vi "DueDACtoAURORA_MM.vi"() -> ()   [LabVIEW 2011]
uses:
  <vilib>/rvi/FXPMathLib/FxpSub/subVIs/nifxpmath_Sub_SimConfig.ctl
  <vilib>/fxp/LVFixedPointQuantizationPolicyTypeDef.ctl
  <vilib>/fxp/LVFixedPointOverflowPolicyTypeDef.ctl
  <vilib>/rvi/FXPMathLib/FxpDiv/subVIs/nifxpmath_Div_SimConfig.ctl
  <vilib>/rvi/interface/RandomDataEmulation/nirviRandomDataFPGAFIFO.vi
  <vilib>/rvi/interface/RandomDataEmulation/niFpgaRandomDataHandleErrors.vi
  <vilib>/rvi/eio/common/nirviEmuTemplateMethod_errors.vi
  <vilib>/rvi/FXPMathLib/FxpSub/simVIs/DllFxpSubTemp_sub.vi
  <vilib>/rvi/FXPMathLib/FxpDiv/simVIs/DllFxpDivTemp_sub.vi
  <vilib>/rvi/DataTransferAndStorage/Container/XNode/niFpgaContainer.xnode
  <vilib>/rvi/interface/RandomDataEmulation/nirviRandomDataFpgaReadWriteTemplate.vi
  <vilib>/eio/EIONode/EIONode.xnode
  <vilib>/rvi/FXPMathLib/FxpAdd/XNode/nifxpmath_Add.xnode
  <vilib>/rvi/FXPMathLib/FxpMul/XNode/nifxpmath_Multiplier.xnode
  <vilib>/rvi/Analysis/measure/butterworth/XNode/niFpgaButterworthFilter.xnode
  <vilib>/rvi/Analysis/common/FxpNativeNode/niFpgaFxpNative.xnode
  <vilib>/rvi/FXPMathLib/FxpSub/XNode/nifxpmath_Sub.xnode
  <vilib>/rvi/FXPMathLib/FxpDiv/XNode/nifxpmath_Div.xnode
  <vilib>/rvi/FXPMathLib/sim/FxpSim.dll
panel:
  in  "N or torque (V)\noutput":bool
  out "non offset torque":fxp<+/-,23,1>
  out "torque to R2":fxp<+/-,23,2>
  out "torque (Nm)":fxp<+/-,23,2>
  in  "torque offset (V)":fxp<+/-,23,2>
  in  "V/Nm":fxp<+/-,21,6>=-17.579986572265625
  out "MM force":fxp<+/-,20,4>
  out "FV gain":fxp<+/-,17,2>
  out "ML/s":fxp<+/-,20,11>
  in  "Velocity filter settings":i16(ring)=1 items=["No filter", "20 Hz Lowpass", "40 Hz  Lowpass", "60 Hz Lowpass"]
  in  "V to ML":fxp<+,15,3>=0.14501953125
  out "length out reset":fxp<+/-,17,10>
  in  "Reset Mode":bool=TRUE
  out "filtered force":fxp<+/-,30,9>
  out "raw force":fxp<+/-,26,5>
  in  "length offset (V)":fxp<+/-,12,5>
  in  "Gandalf volts/rad":fxp<+/-,17,6>=12.33984375
  in  "abs length limit (V)":fxp<+/-,12,5>=9.0
  out "offset dac":fxp<+/-,27,6>
  out "Mujoco\nmuscle length\nscaled 0.145 ML/V":fxp<+/-,26,5>
  in  "DU dac gain":fxp<+/-,16,2>=1.25
  in  "DU dac\noffset":fxp<+/-,16,1>=-0.555999755859375
  out "from DUE dac0":fxp<+/-,26,5>
  out "loop time (ticks)":u32
  out "length out (V)":fxp<+/-,17,10>
  in  "Reset":bool=TRUE
  in  "Timeout":i32
  out "Full Flag\nTimed Out?":bool
  # "NOTE: Dac output has\nto be truncated so only\n2 digits of precision due\nto uncertainty of the rest."
  # "Convert 0-2.2V output to full muscle strain 0.32 ML\nEstimated by muscle dL required to make joints 180"
  # "Gain and offset to compensate for limitations of Arduino DUE\nDAC"
  # "<--Negate depending\non R2D2 direction needed"
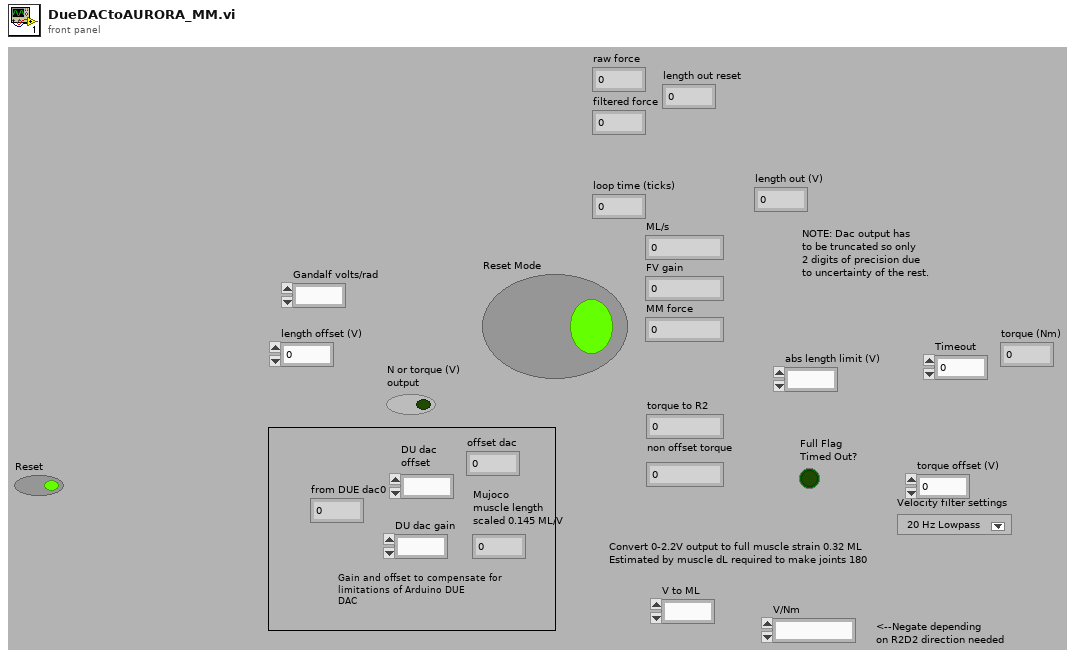
[diagram p1: front panel]
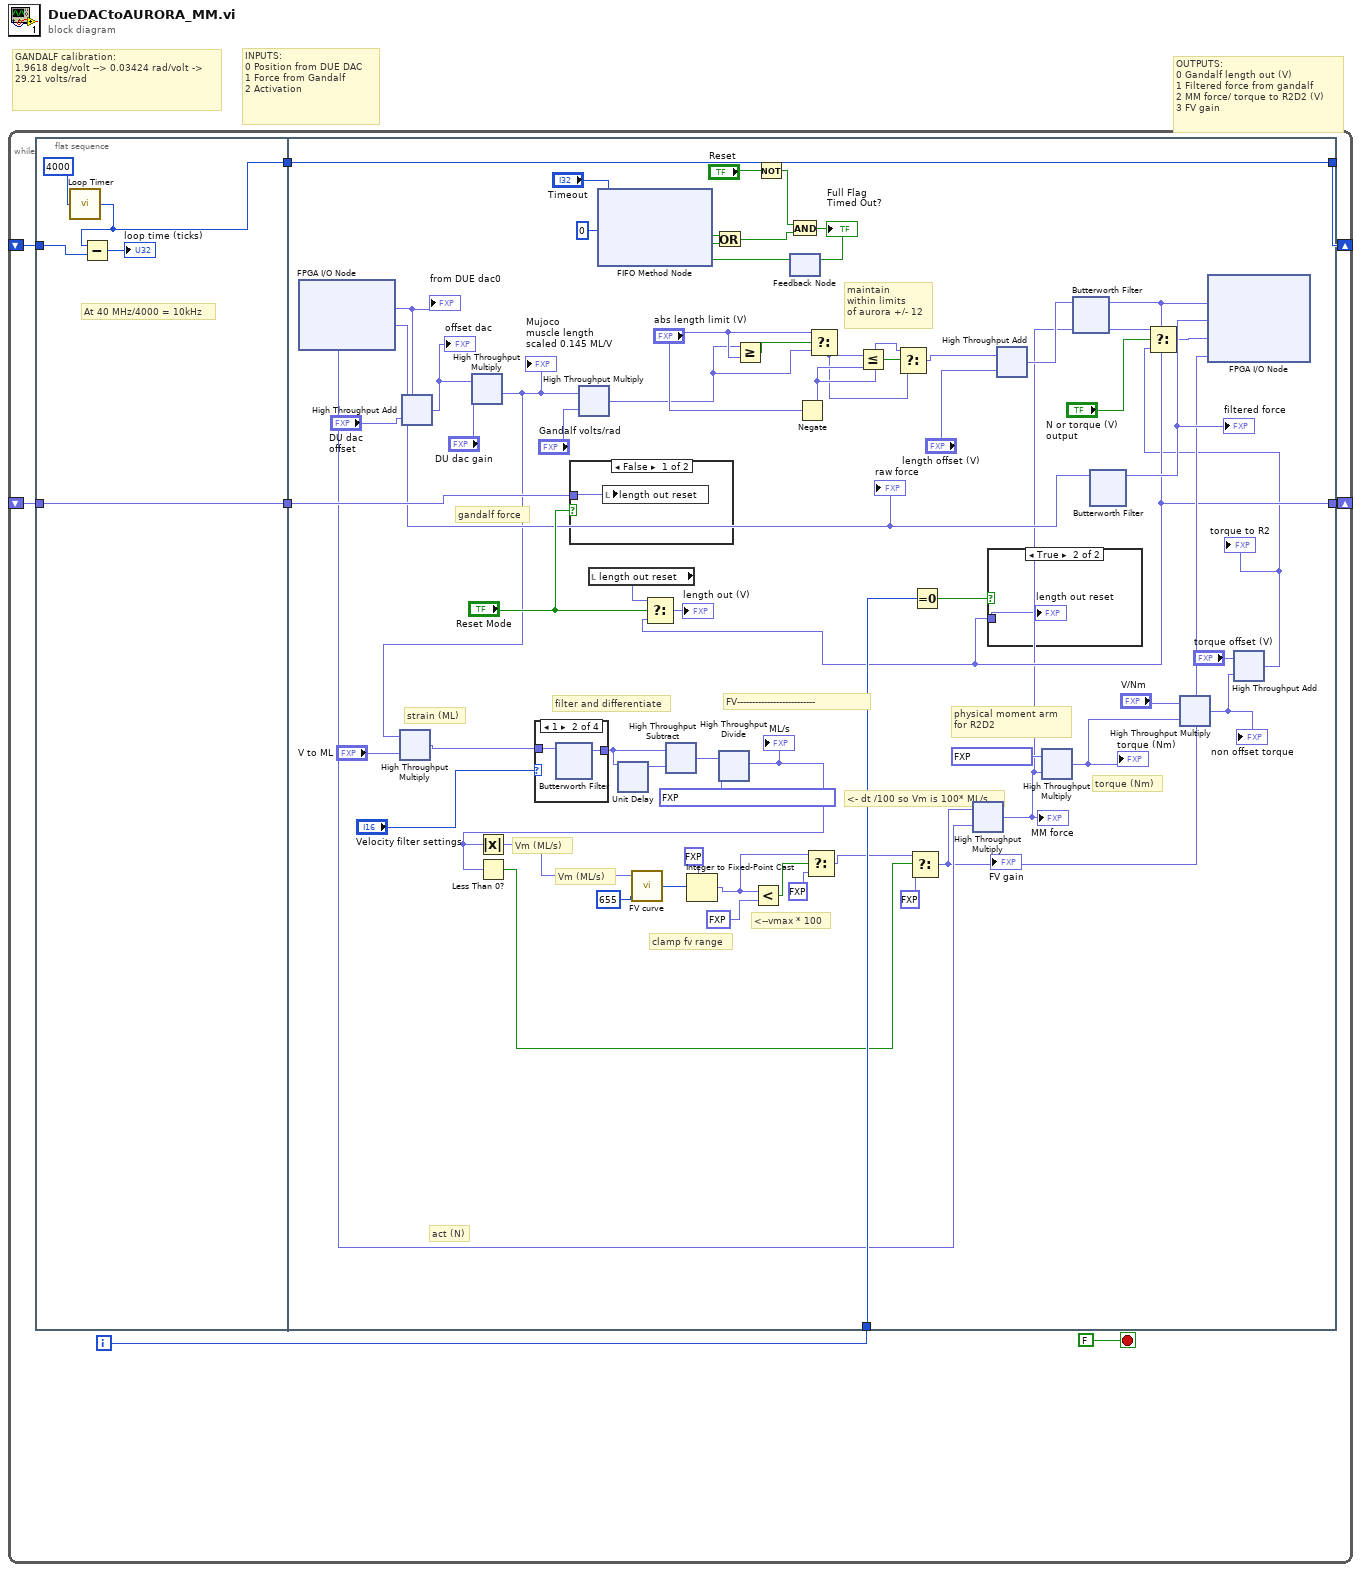
[diagram p0: block diagram]
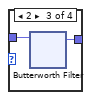
[diagram p3: hidden frame]
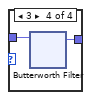
[diagram p4: hidden frame]
diagram:
  # "GANDALF calibration:\n1.9618 deg/volt --> 0.03424 rad/volt ->\n29.21 volts/rad"
  # "INPUTS:\n0 Position from DUE DAC\n1 Force from Gandalf\n2 Activation"
  # "OUTPUTS:\n0 Gandalf length out (V)\n1 Filtered force from gandalf\n2 MM force/ torque to R2D2 (V)\n3 FV gain"
  n1 = while {
    shift-right: [w7] -> _
    shift-left: _ -> [w5]
    shift-right: [w4] -> _
    shift-left: _ -> [w2]
    i -> [w1]
    stop <- FALSE stop-if-true
    n2 = flat-sequence {
      tunnel: [w11] -> w6
      tunnel: w5 -> [w12]
      tunnel: [w9] -> w3
      tunnel: w2 -> [w9]
      tunnel: [w69] -> w7
      tunnel: w6 -> [w69]
      tunnel: [w18] -> w4
      tunnel: w3 -> [w54]
      tunnel: w1 -> [w50]
      frame #0 {
        # "At 40 MHz/4000 = 10kHz"
        n3 = call "Loop Timer"("Count(Ticks)"=u32 4000) -> ("Tick Count(Ticks)"=w11:u32)
        n4 = Subtract(x=w11, y=w12) -> (x-y=→"loop time (ticks)":u32)
      }
      frame #1 {
        # "<--vmax * 100"
        # "clamp fv range"
        # "Vm (ML/s)"
        # "<- dt /100 so Vm is 100* ML/s"
        # "physical moment arm\nfor R2D2"
        # "torque (Nm)"
        # "gandalf force"
        # "act (N)"
        # "filter and differentiate"
        # "FV--------------------------"
        # "Vm (ML/s)"
        # "strain (ML)"
        # "maintain \nwithin limits\nof aurora +/- 12"
        n5 = xnode "FPGA I/O Node"() -> ("Mod2/AI0"=w20:fxp<+/-,26,5>, "Mod2/AI1"=w48:fxp<+/-,26,5>, "Mod2/AI2"=w27:fxp<+/-,26,5>)  [unwired: 3 in, 3 out]
        "from DUE dac0" <- w20
        "raw force" <- w48
        n6 = xnode "High Throughput Add"("x"=w20, "y"="DU dac\noffset") -> ("x+y"=w60:fxp<+/-,26,5>)
        "offset dac" <- w60
        n7 = xnode "High Throughput Multiply"("x"=w60, "y"="DU dac gain") -> ("x*y"=w38:fxp<+/-,26,5>)
        "Mujoco\nmuscle length\nscaled 0.145 ML/V" <- w38
        n8 = xnode "High Throughput Multiply"("x"=w38, "y"="V to ML") -> ("x*y"=w39:fxp<+/-,25,2>)
        n9 = case shown="1" "Velocity filter settings" {
          tunnel: [w91 w93 w102 w111] -> w44
          tunnel: w39 -> [w91 w92 w101 w110]
          frame 0, Default {
            # "no filter"
          }
          frame 1 {
            n10 = xnode "Butterworth Filter"("input data"=w92) -> ("output data"=w93:fxp<+/-,25,2>)  [unwired: 2 in]
          }
          frame 2 {
            n11 = xnode "Butterworth Filter"("input data"=w101) -> ("output data"=w102:fxp<+/-,25,2>)  [unwired: 2 in]
          }
          frame 3 {
            n12 = xnode "Butterworth Filter"("input data"=w110) -> ("output data"=w111:fxp<+/-,25,2>)  [unwired: 2 in]
          }
        }
        n13 = case shown="False" "Reset Mode" {
          tunnel: w54 -> [w184 _]
          frame False {
            n14 = local write "length out reset"(w184) -> ()
          }
          frame True {
          }
        }
        n15 = xnode "High Throughput Multiply"("x"=w38, "y"="Gandalf volts/rad") -> ("x*y"=w58:fxp<+/-,12,5>)
        n16 = local read "length out reset"() -> (w49:fxp<+/-,17,10>)
        n17 = xnode ("FIFO Method Node")("Element"=i16 0, "Timeout"="Timeout") -> ("Timed Out?"=w75:bool)  [unwired: 1 in, 1 out]
        n18 = xnode ("Unit Delay")("input"=w44) -> ("output"=w46:fxp<+/-,25,2>)  [unwired: 2 in]
        n19 = xnode "High Throughput Subtract"("x"=w44, "y"=w46) -> ("x-y"=w43:fxp<+/-,30,1>)
        n20 = xnode "High Throughput Divide"("x"=w43, "y"=fxp<+/-,32,1> 9.997747838497162e-07) -> ("x/y"=w42:fxp<+/-,20,11>)
        "ML/s" <- w42
        n21 = Absolute Value(x=w42) -> (abs(x)=w29:fxp<+,20,11>)
        n22 = Less Than 0?(x=w42) -> (x < 0?=w41:bool)
        n23 = call "FV curve"("address"=w29, "fractional index (x 2^16)"=u16 655) -> ("data out"=w31:i16)  [unwired: 7 in]
        n24 = Integer to Fixed-Point Cast(fixed-point type=fxp<+/-,16,1> 0.0 ("fixed-point"), integer=w31) -> (fixed-point=w23:fxp<+/-,16,1>)
        n25 = Greater Or Equal?(x=w58, y="abs length limit (V)") -> (x >= y?=w67:bool)
        n26 = Less?(x=w23, y=fxp<+/-,20,11> 900.0 ("x/y")) -> (x < y?=w24:bool)
        n27 = Not(x="Reset") -> (.not. x?=w73:bool)
        n28 = feedback #1() -> (w70:bool)  [unwired: 1 in]
        n29 = Or(x=w70, y=w75) -> (x .or. y?=w72:bool)
        n30 = And(x=w73, y=w72) -> (x .and. y?=w71:bool)
        "Full Flag\nTimed Out?" <- w71
        n31 = feedback-in #1(w71) -> ()
        n32 = Negate(x="abs length limit (V)") -> (-x=w64:fxp<+/-,13,6>)
        n33 = Select(t=w23, s=w24, f=fxp<+/-,16,1> 0.0) -> (s? t:f=w21:fxp<+/-,16,1>)
        n34 = Select(t="abs length limit (V)", s=w67, f=w58) -> (s? t:f=w63:fxp<+/-,12,5>)
        n35 = Less Or Equal?(x=w63, y=w64) -> (x <= y?=w65:bool)
        n36 = Select(t=w64, s=w65, f=w63) -> (s? t:f=w56:fxp<+/-,13,6>)
        n37 = Select(t=w21, s=w41, f=fxp<+/-,17,2> 1.0) -> (s? t:f=w26:fxp<+/-,17,2>)
        "FV gain" <- w26
        n38 = Equal To 0?(x=w50) -> (x = 0?=w51:bool)
        n39 = xnode "High Throughput Multiply"("x"=w26, "y"=w27) -> ("x*y"=w15:fxp<+/-,20,4>)
        "MM force" <- w15
        n40 = xnode "High Throughput Add"("x"=w56, "y"="length offset (V)") -> ("x+y"=w19:fxp<+/-,12,5>)
        n41 = xnode "High Throughput Multiply"("x"=fxp<+/-,21,6> 0.02001953125, "y"=w15) -> ("x*y"=w35:fxp<+/-,23,2>)
        "torque (Nm)" <- w35
        n42 = xnode "Butterworth Filter"("input data"=w19) -> ("output data"=w18:fxp<+/-,16,9>)  [unwired: 2 in]
        n43 = Select(t=w49, s="Reset Mode", f=w18) -> (s? t:f=→"length out (V)":fxp<+/-,17,10>)
        n44 = case shown="True" w51 {
          tunnel: w18 -> [_ w183]
          frame False {
          }
          frame True {
            "length out reset" <- w183
          }
        }
        n45 = xnode "Butterworth Filter"("input data"=w48) -> ("output data"=w55:fxp<+/-,30,9>)  [unwired: 2 in]
        "filtered force" <- w55
        n46 = xnode "High Throughput Multiply"("x"="V/Nm", "y"=w35) -> ("x*y"=w33:fxp<+/-,23,1>)
        "non offset torque" <- w33
        n47 = xnode "High Throughput Add"("x"="torque offset (V)", "y"=w33) -> ("x+y"=w16:fxp<+/-,23,2>)
        "torque to R2" <- w16
        n48 = Select(t=w15, s="N or torque (V)\noutput", f=w16) -> (s? t:f=w17:fxp<+/-,25,4>)
        n49 = xnode "FPGA I/O Node"("Mod1/AO0"=w18, "Mod1/AO1"=w55, "Mod1/AO2"=w17, "Mod1/AO3"=w26) -> ()  [unwired: 4 in, 4 out]
      }
    }
  }
